vi "testSentTelToTcpClientAtDiffRates.vi"(8 "error in (no error)":errorcluster) -> (0 "error out":errorcluster)   [LabVIEW 2018]
uses:
  <vilib>/addons/_JKI Toolkits/Caraya/classes/Assert/Assert Equal Value_Variant.vi
  <vilib>/addons/_JKI Toolkits/Caraya/classes/Test/Test.lvclass
  src/TcpServer/TcpServer.lvclass
  <vilib>/addons/_JKI Toolkits/Caraya/classes/Assert/Assert.lvclass
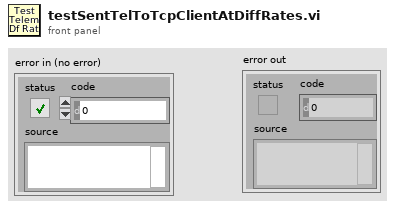
[diagram p1: front panel]
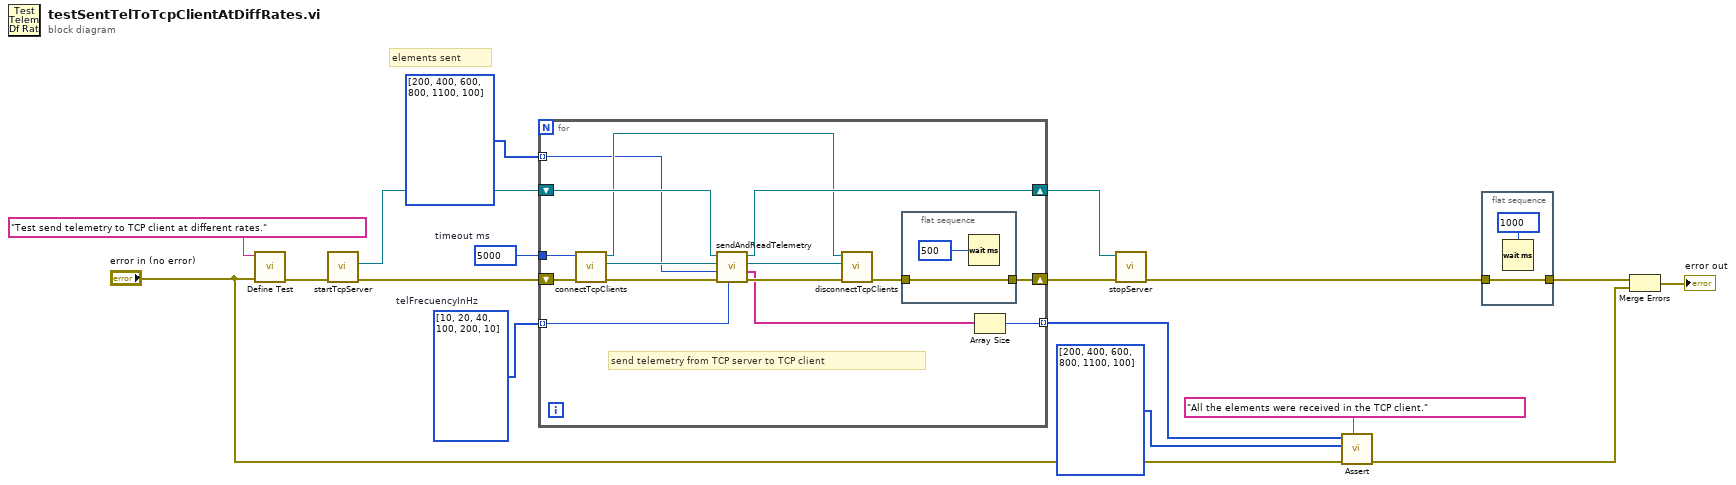
[diagram p0: block diagram]
diagram:
  w3 = u32[] [10, 20, 40, 100, 200, 10]  # telFrecuencyInHz
  w7 = 5000  # timeout ms
  # "elements sent"
  n1 = call <vilib>:"Define Test.vi"("error in (no error)"="error in (no error)", "Label (VI Title)"="Test send telemetry to TCP client at different rates.") -> ("error out"=w16:errorcluster)  [unwired: 9 in]
  n2 = call "startTcpServer.vi"("error in (no error)"=w16) -> ("error out"=w6:errorcluster, "TcpServer out"=w9:refnum<class "TcpServer.lvclass">)  [unwired: 8 in, 1 out]
  n3 = for {
    shift-right: [w19] -> w15
    shift-left: w6 -> [w32]
    shift-right: [w28] -> w14
    shift-left: w9 -> [w31]
    tunnel: i32[] [200, 400, 600, 800, 1100, 100] -> [w25] mode=indexing
    tunnel: w7 -> [w26]
    tunnel: [w21] -> w4 mode=indexing
    tunnel: w3 -> [w20] mode=indexing
    # "send telemetry from TCP server to TCP client"
    n4 = call "connectTcpClients.vi"("error in (no error)"=w32, "timeout ms"=w26) -> ("error out"=w24:errorcluster, "tel connection ID out"=w30:refnum<k5>, "cmd connection ID out"=w27:refnum<k5>)  [unwired: 7 in]
    n5 = call "sendAndReadTelemetry.vi"("telFrecuencyInHz (10)"=w20, "error in (no error)"=w24, "numPackets (50)"=w25, "tel connection in"=w30, "TcpServer out"=w31) -> ("error out"=w23:errorcluster, "telemetry received"=w22:string[], "tel connection out"=w29:refnum<k5>, "tcpServer out"=w28:refnum<class "TcpServer.lvclass">)  [unwired: 3 in]
    n6 = call "disconnectTcpClients.vi"("error in (no error)"=w23, "tel connection ID in"=w29, "cmd connection ID in"=w27) -> ("error out"=w18:errorcluster)  [unwired: 8 in]
    n7 = flat-sequence {
      tunnel: [w33] -> w19
      tunnel: w18 -> [w33]
      frame #0 {
        n8 = Wait (ms)(milliseconds to wait=u32 500) -> ()  [unwired: 1 out]
      }
    }
    n9 = Array Size(array=w22) -> (size(s)=w21:i32)
  }
  n10 = call "stopServer.vi"("error in (no error)"=w15, "tcpServer in"=w14) -> ("error out"=w1:errorcluster)  [unwired: 8 in, 1 out]
  n11 = call-poly <vilib>:"Assert.vi"("Label"="All the elements were received in the TCP client.", "error in (no error)"="error in (no error)", "Y"=i32[] [200, 400, 600, 800, 1100, 100], "X"=w4) -> ("error out"=w11:errorcluster)  [unwired: 7 in]
  n12 = flat-sequence {
    tunnel: [w35] -> w2
    tunnel: w1 -> [w35]
    frame #0 {
      n13 = Wait (ms)(milliseconds to wait=u32 1000) -> ()  [unwired: 1 out]
    }
  }
  n14 = Merge Errors(w2, w11) -> (→"error out":errorcluster)
